vi "dsdll_close.vi"(8 "error in":errorcluster, 11 "dsdll instance in":T1={"dsdll path"=path "E:/LVprog/DirectSoundDLL/dsdll.dll", "dsdll handle"=[], "output devices"=[], "capture devices"=[]}) -> (0 "error out":errorcluster, 3 "dsdll instance out":T1)   [LabVIEW 2020, in "dsdll.lvlib"]
doc: "Call this to close DSDLL instance. This VI tries to close it even if there is error at error input. If some playback or capture is in progress it will be terminated."
uses:
  dsdll.lvlib
  dsdll_instance.ctl
  dsdll_device_record.ctl
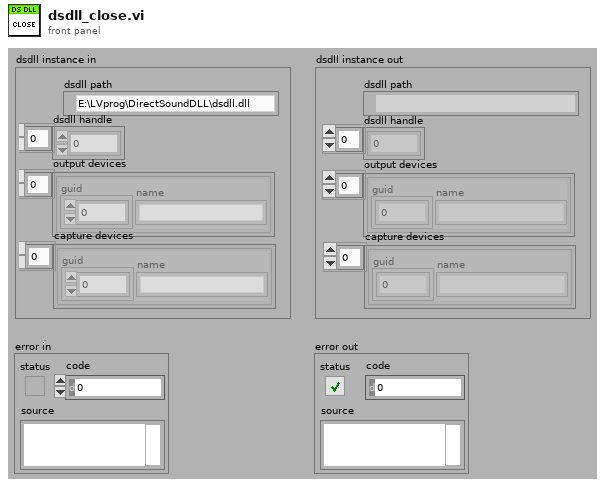
[diagram p1: front panel]
types:
  T1 = typedef "dsdll.lvlib/dsdll_instance.ctl" = cluster{"dsdll path":path, "dsdll handle":u8[], "output devices":T2[], "capture devices":T2[]}
  T2 = typedef "dsdll.lvlib/dsdll_device_record.ctl" = cluster{"guid":u8[], "name":string}
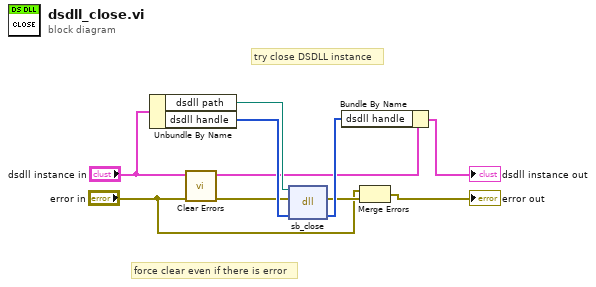
[diagram p0: block diagram]
diagram:
  # "force clear even if there is error"
  # "try close DSDLL instance"
  n1 = Unbundle By Name("dsdll instance in") -> ("dsdll path"=w7:path, "dsdll handle"=w6:u8[])
  n2 = call <vilib>:"Clear Errors.vi"("error in (no error)"="error in") -> ("error out"=w4:errorcluster)  [unwired: 5 in, 1 out]
  n3 = dll-call lib="dsdll.dll" fn="sb_close" ("sb_get_handle_size()")(path in=w7, error in=w4, "handle"=w6) -> (error out=w3:errorcluster, "handle"=w5:u8[])  [unwired: 2 in, 1 out]
  n4 = Bundle By Name(cluster="dsdll instance in", "dsdll handle"=w5) -> (→"dsdll instance out":T1)
  n5 = Merge Errors("error in", w3) -> (→"error out":errorcluster)
